vi "SetByteOrder.vi"(8 "Error In":errorcluster, 10 "Byte Order":T1, 11 "Keithley 6485 In":refnum<visa-resource-name>) -> (0 "Error Out":errorcluster, 3 "Keithley 6485 Out":refnum<visa-resource-name>)   [LabVIEW 2012, in "Keithley-6485.lvlib"]
uses:
  Keithley-6485.lvlib
  Controls/ByteOrder.ctl
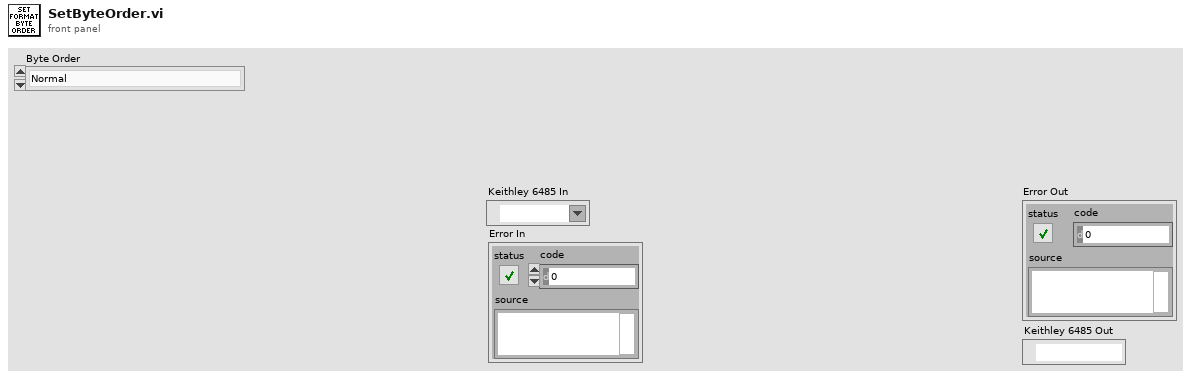
[diagram p1: front panel]
types:
  T1 = typedef "Keithley-6485.lvlib/ByteOrder.ctl" = enum16{"Normal", "Swapped"}
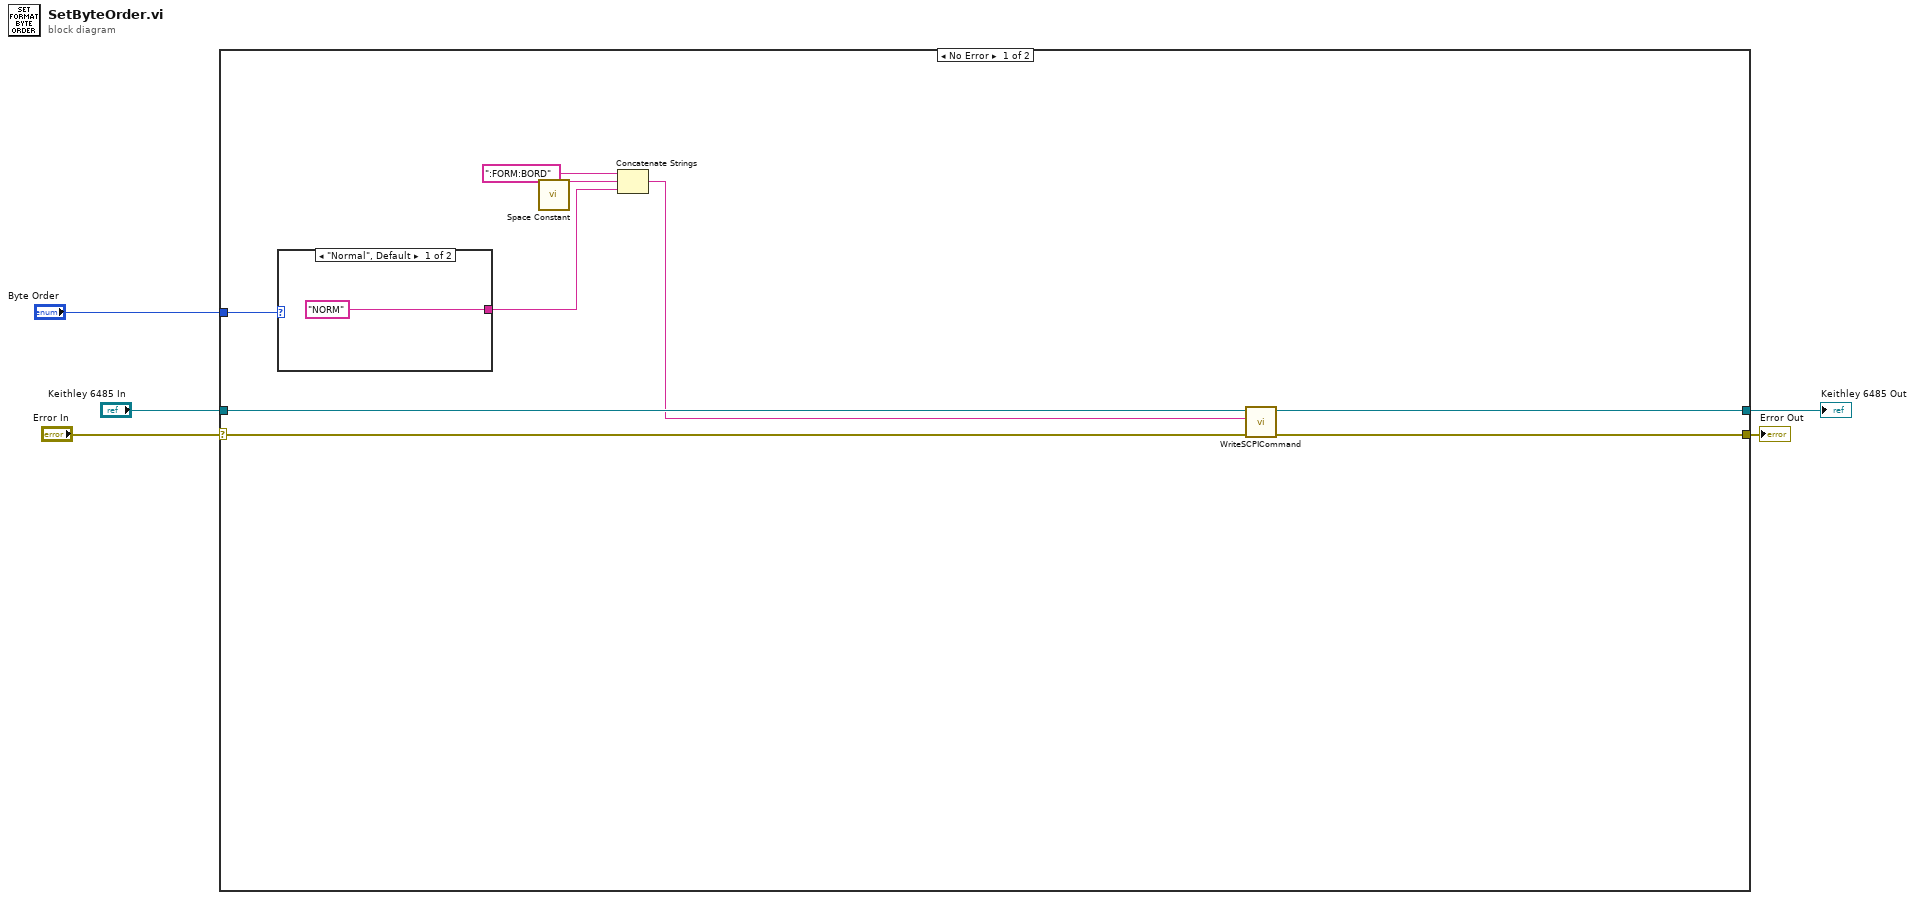
[diagram p0: block diagram]
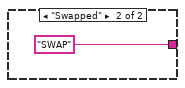
[diagram p2: hidden frame]
diagram:
  n1 = case shown="No Error" "Error In" {
    selector: "Error In" -> [w9 w17]
    tunnel: "Keithley 6485 In" -> [w8 w18]
    tunnel: [w10 w17] -> w3
    tunnel: [w11 w18] -> w2
    tunnel: "Byte Order" -> [w6 _]
    frame No Error {
      n2 = case shown="\"Normal\", Default" w6 {
        tunnel: ["NORM" "SWAP"] -> w12
        frame "Normal", Default {
        }
        frame "Swapped" {
        }
      }
      n3 = call <vilib>:"Space Constant.vi"() -> ("String"=w13:string)
      n4 = Concatenate Strings(":FORM:BORD", w13, w12) -> (w7:string)
      n5 = call "WriteSCPICommand.vi"("Error In"=w9, "SCPI Command"=w7, "Keithley 6482 In"=w8) -> ("Error Out"=w10:errorcluster, "Keithley 6482 Out"=w11:refnum<visa-resource-name>)  [unwired: 7 in]
    }
    frame Error {
    }
  }
  "Error Out" <- w3
  "Keithley 6485 Out" <- w2
